vi "getMessage.vi"(8 "error in (no error)":errorcluster, 10 "message_end":T1, 11 "tcpDevice in":refnum<class "tcpDevice.lvclass">) -> (0 "error out":errorcluster, 1 "timeout":bool, 2 "Message":string, 3 "tcpDevice out":refnum<class "tcpDevice.lvclass">)   [LabVIEW 2016, in "tcpDevice.lvclass"]
uses:
  tcpDevice.lvclass
  typedefs/messageEnd.ctl
  tcpDevice.lvclass/tcpDevice.ctl
  ts_labview_tcp/TCPClient/TCPClient.lvclass
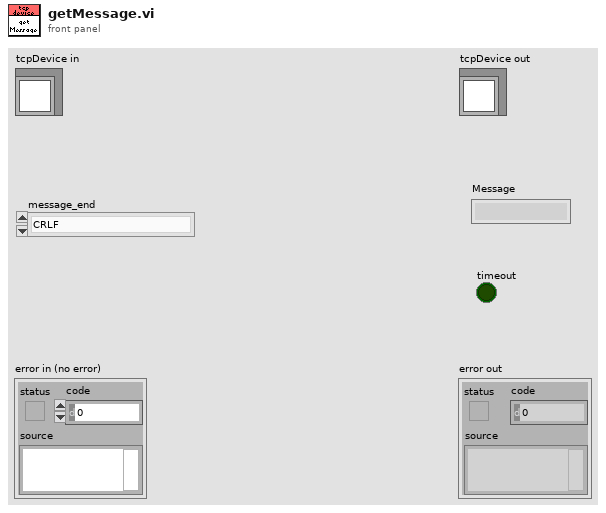
[diagram p1: front panel]
types:
  T1 = typedef "messageEnd.ctl" = enum16{"CRLF"}
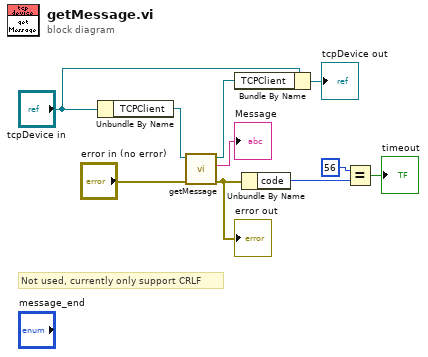
[diagram p0: block diagram]
diagram:
  # "Not used, currently only support CRLF"
  n1 = Unbundle By Name("tcpDevice in") -> ("TCPClient"=w8:refnum<class "TCPClient.lvclass">)
  n2 = call-dynamic "getMessage.vi"("error in (no error)"="error in (no error)", "TCPClient in"=w8) -> ("error out"=w4:errorcluster, "String"=→"Message":string, "TCPClient out"=w7:refnum<class "TCPClient.lvclass">)  [unwired: 7 in]
  "error out" <- w4
  n3 = Bundle By Name(cluster="tcpDevice in", "TCPClient"=w7) -> (→"tcpDevice out":refnum<class "tcpDevice.lvclass">)
  n4 = Unbundle By Name(w4) -> ("code"=w3:i32)
  n5 = Equal?(x=56, y=w3) -> (x = y?=→"timeout":bool)
